vi "Simulate.vi"() -> ()   [LabVIEW 2018, in "Serial.lvlib"]
uses:
  Serial.lvlib
  <vilib>/Platform/TimedLoop/XDataNode/timing_clust.ctl
  <vilib>/Platform/TimedLoop/XDataNode/nitl_modes.ctl
  <vilib>/Platform/TimedLoop/XDataNode/wakeup.ctl
  <vilib>/Instr/_visa.llb/VISA Configure Serial Port (Instr).vi
  <vilib>/platform/TimedLoop/XDataNode/XDataNode.xnode
  <vilib>/Platform/TimedLoop/XDataNode/XDNodeRunTimeDep.lvlib
panel:
  in  "?":enum32{"Simulation", "Communication", "Loop"}(tab)
  out "Mean":dbl
  in  "Simulate Output":bool
  out "Counter":u32
  out "Signal":dynamicdata(graph)
  in  "Amplitude":dbl(slide)=10.0 scale=0.0..10.0
  in  "Frequency":dbl(slide)=40.39408866995074 scale=0.0..100.0
  in  "Serial port":refnum<visa-resource-name>="COM1"
  in  "Frequency":dbl(slide) scale=1.0..100.0
  in  "Stop":bool
  out "Counter":i32
  out "Interval":i64
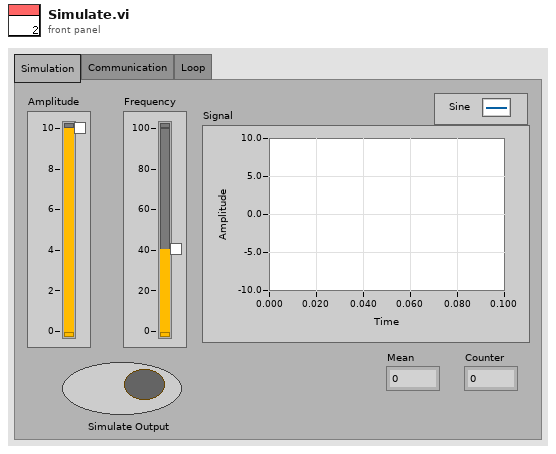
[diagram p1: front panel]
types:
  T1 = typedef "XDNodeRunTimeDep.lvlib/timing_clust.ctl" = cluster{"Expected End [f-1]":u64, "Actual End [f-1]":u64, "Finished Late? [f-1]":bool, "Expected End [i-1]":u64, "Actual End [i-1]":u64, "Finished Late? [i-1]":bool, "Expected Start [i]":u64, "Actual Start [i]":u64, "Expected Start [f]":u64, "Actual Start [f]":u64, "Source Name":string, "Structure Name":string, "Period":i64, "Deadline":i64, "Offset":i64, "Start":i64, "Priority":i32, "Timeout":i32, "Mode":T2, "Wakeup Reason":T3, "Error":errorcluster, "Source Type":string, "Secondary Source Type":string, "Global End Time":u64, "Global Start Time":u64, "Frame Duration":u64, "Iteration Duration":u64, "Assigned CPU":i32, "I/O Scan Engine Mode":u32}
  T2 = typedef "XDNodeRunTimeDep.lvlib/nitl_modes.ctl" = enum32{"No Change", "Process missed periods, maintain original phase", "Discard missed periods, maintain original phase", "Process missed periods, ignore original phase", "Discard missed periods, ignore original phase"}
  T3 = typedef "XDNodeRunTimeDep.lvlib/wakeup.ctl" = enum32{"Normal", "Aborted", "Asynchronous wakeup", "Timing source error", "Timed loop error", "Timeout"}
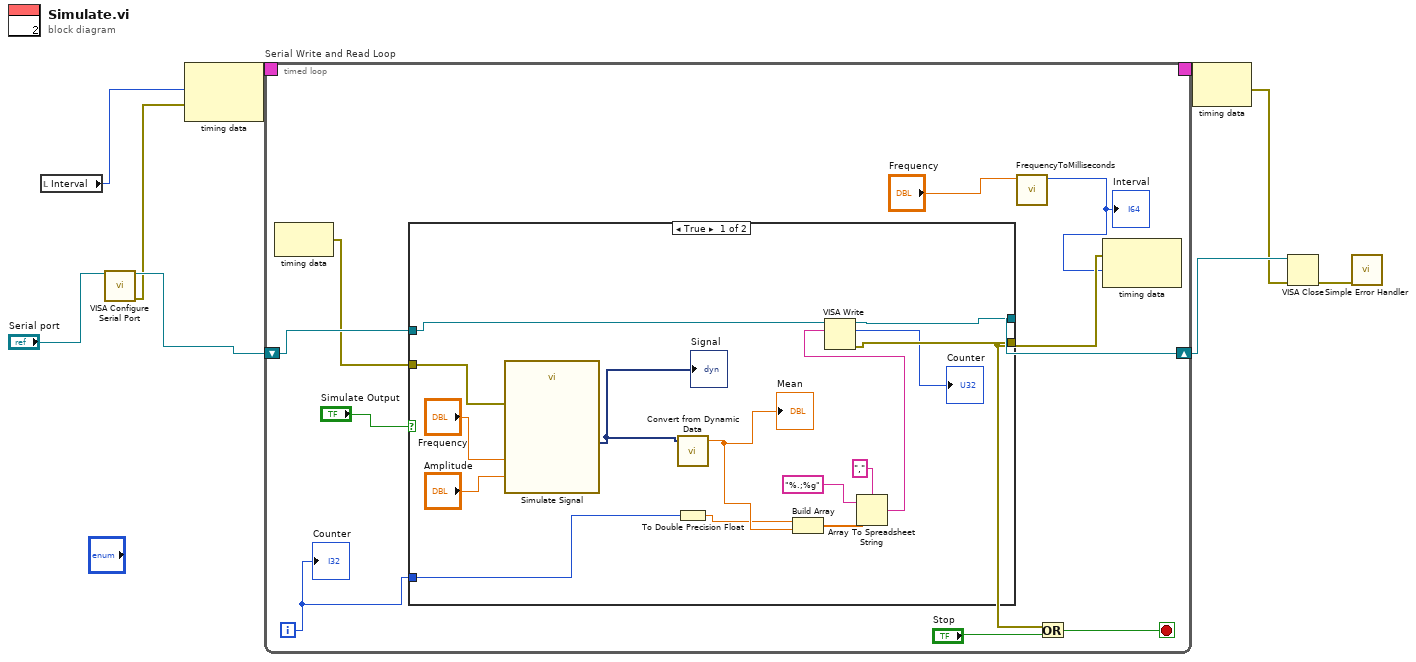
[diagram p0: block diagram]
diagram:
  n1 = local read "Interval"() -> (w1:i64)
  n2 = call-poly "VISA Configure Serial Port"("VISA resource name"="Serial port") -> ("VISA resource name out"=w6:refnum<visa-resource-name>, "error out"=w5:errorcluster)  [unwired: 9 in, 4 out]
  n3 = node-c288(w1, w5) -> (w8:T1)
  n4 = timed-loop "Serial Write and Read Loop" {
    timing: w8 -> [_]
    timing-out: [_] -> w7
    shift-right: [w16] -> w4
    shift-left: w6 -> [w17]
    i -> [w13]
    stop <- w12 stop-if-true
    n5 = node-c288() -> (w14:errorcluster)  [unwired: 1 in]
    n6 = case shown="True" "Simulate Output" {
      tunnel: [w31 w36] -> w16
      tunnel: [w32 w35] -> w15
      tunnel: w17 -> [w29 w36]
      tunnel: w14 -> [w26 w35]
      tunnel: w13 -> [w21 _]
      frame True {
        n7 = call "Simulate Signal"("Frequency"="Frequency", "Amplitude"="Amplitude", "error in (no error)"=w26) -> ("Sine"=w24:dynamicdata)  [unwired: 3 in, 9 out]
        "Signal" <- w24
        n8 = call "Convert from Dynamic Data"("Dynamic Data Type"=w24) -> ("Scalar"=w23:dbl)  [unwired: 3 in]
        "Mean" <- w23
        n9 = To Double Precision Float(number=w21) -> (double precision float=w22:dbl)
        n10 = Build Array(w22, w23) -> (w25:dbl[])
        n11 = Array To Spreadsheet String(delimiter (Tab)=",", array=w25, 3:"%.;%g" ("format string")) -> (spreadsheet string=w20:string)
        n12 = VISA Write(VISA resource name=w29, write buffer=w20) -> (VISA resource name out=w31:refnum<visa-resource-name>, return count=→"Counter":u32, error out=w32:errorcluster)  [unwired: 1 in]
      }
      frame False {
      }
    }
    n13 = call "FrequencyToMilliseconds.vi"("Frequency"="Frequency") -> ("Numeric"=w10:i64)  [unwired: 10 in]
    "Interval" <- w10
    n14 = Or(x=w15, y="Stop") -> (x .or. y?=w12:bool)
    n15 = node-c288(w15, w10) -> ()  [unwired: 1 out]
    "Counter" <- w13
  }
  n16 = node-c288(w7) -> (w3:errorcluster)
  n17 = VISA Close(VISA resource name=w4, error in (no error)=w3) -> (error out=w2:errorcluster)
  n18 = call <vilib>:"Simple Error Handler.vi"("error in (no error)"=w2) -> ()  [unwired: 1 in, 8 out]
